vi "SENS_CORR_EXT_PORT_TIME.vi"(0 "VISA IN":refnum<visa-resource-name>, 1 "Port":i32, 2 "Port Ext. (sec)":i32, 5 "error in":errorcluster, 7 "Channel":i32) -> (14 "VISA Out":refnum<visa-resource-name>, 19 "error out":errorcluster)   [LabVIEW 2018, in "PNA-X.lvlib"]
doc: "SENSe<cnum>:CORRection:EXTension:PORT<pnum>[:TIME] <num> \n1706\n\n(Read-Write) Sets the extension value at the specified port. Must also set SENS:CORR:EXT ON. \nNote: This command affects ALL measurements on the specified channel. \nParameters \n<cnum> Any existing channel number. If unspecified, value is set to 1 \n<pnum> Port Number that will receive the extension. If unspecified, value is set to 1. \n<num> The port extension in seconds; may include suffix. Choose a number between: \n-1E18 and 1E18 \nExamples SENS:CORR:EXT:PORT 2MS \nsense2:correction:extension:port2 .00025 \nQuery Syntax SENSe<cnum>:CORRection:EXTension:PORT<pnum> [:TIME]? \nReturn Type Numeric \nDefault 0"
uses:
  PNA-X.lvlib
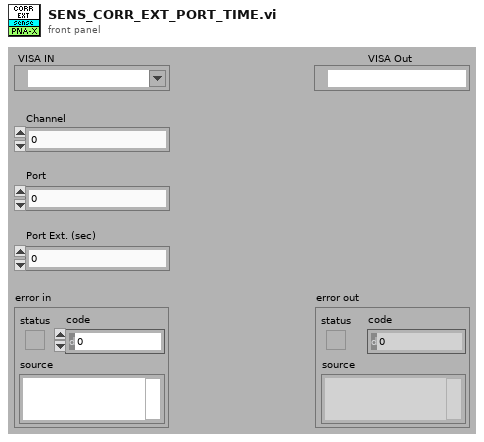
[diagram p1: front panel]
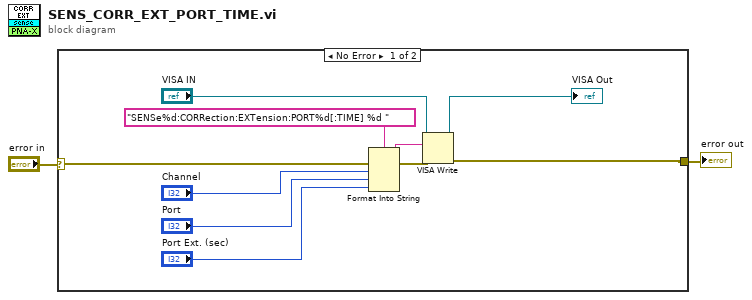
[diagram p0: block diagram]
diagram:
  n1 = case shown="No Error" "error in" {
    selector: "error in" -> [w12 w13]
    tunnel: [w7 w13] -> w1
    frame No Error {
      n2 = Format Into String(format string="SENSe%d:CORRection:EXTension:PORT%d[:TIME] %d " ("Cmdline"), error in=w12, "Channel", "Port", "Port Ext. (sec)") -> (resulting string=w10:string, error out=w11:errorcluster)  [unwired: 1 in]
      n3 = VISA Write(VISA resource name="VISA IN", write buffer=w10, error in (no error)=w11) -> (VISA resource name out=→"VISA Out":refnum<visa-resource-name>, error out=w7:errorcluster)  [unwired: 1 out]
    }
    frame Error {
    }
  }
  "error out" <- w1
